vi "testBuildStateStringWithArguments.vi"(8 "error in (no error)":errorcluster, 11 "testStateMachineUtilities in":refnum<class "testStateMachineUtilities.lvclass">) -> (0 "error out":errorcluster, 3 "testStateMachineUtilities out":refnum<class "testStateMachineUtilities.lvclass">)   [LabVIEW 2013, in "testStateMachineUtilities.lvclass"]
uses:
  testStateMachineUtilities.lvclass
  source/State Machine Support API/Support/Trim Whitespace - Inlined.vi
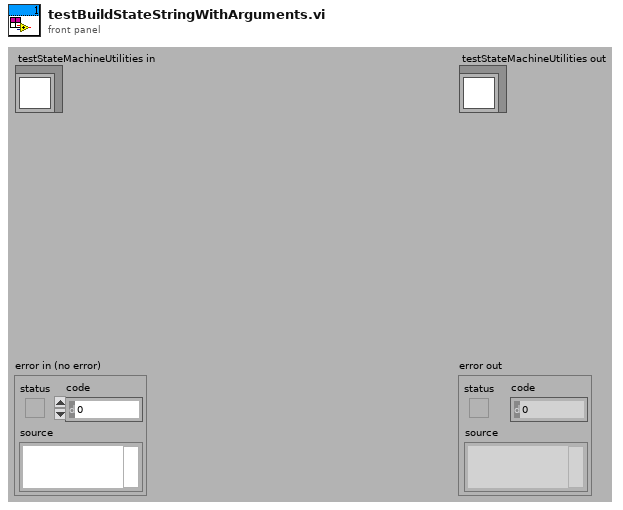
[diagram p1: front panel]
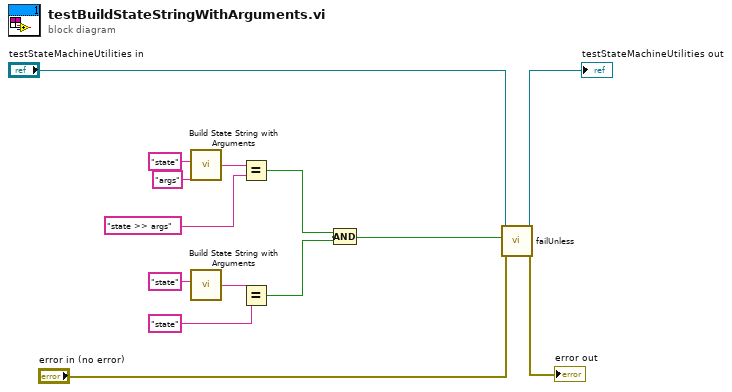
[diagram p0: block diagram]
diagram:
  n1 = call "Build State String with Arguments.vi"("Arguments (\"\")"="args" ("Arguments (\"\")"), "State"="state") -> ("State with Arguments"=w8:string)  [unwired: 4 in]
  n2 = call "Build State String with Arguments.vi"("State"="state") -> ("State with Arguments"=w5:string)  [unwired: 5 in]
  n3 = Equal?(x=w8, y="state >> args" ("Arguments (\"\")")) -> (x = y?=w3:bool)
  n4 = Equal?(x=w5, y="state" ("State")) -> (x = y?=w2:bool)
  n5 = Compound Arithmetic op=AND(w3, w2) -> (w1:bool)
  n6 = call-dynamic "failUnless.vi"("error in (no error)"="error in (no error)", "pass"=w1, "TestCase in"="testStateMachineUtilities in") -> ("error out"=→"error out":errorcluster, "TestCase out"=→"testStateMachineUtilities out":refnum<class "testStateMachineUtilities.lvclass">)  [unwired: 7 in]
